vi "Alarm URL to Tag Name.vi"(11 "alarm URL":string="\\\\Nate-VM-LV2018\\Pfizer_FAST_20190409T090342\\Temperature.Alarms.Temperature:Lo") -> (3 "tag name":string)   [LabVIEW 2021, in "Dynamic Shared Variables.lvlib"]
uses:
  Dynamic Shared Variables.lvlib
  <vilib>/regexp/Match Regular Expression.xnode
panel:
  out "string after last '\\'.":string
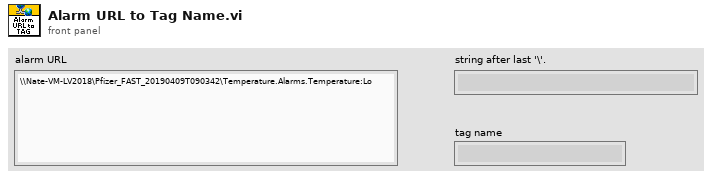
[diagram p1: front panel]
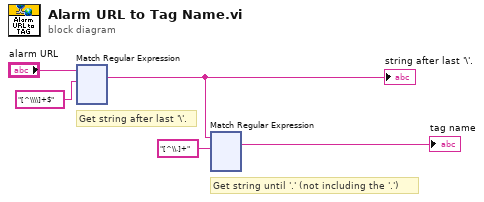
[diagram p0: block diagram]
diagram:
  # "Get string until '.' (not including the '.')"
  # "Get string after last '\\'."
  n1 = xnode "Match Regular Expression"("input string"="alarm URL", "regular expression"="[^\\\\]+$") -> ("whole match"=w3:string)  [unwired: 4 in, 4 out]
  "string after last '\\'." <- w3
  n2 = xnode "Match Regular Expression"("input string"=w3, "regular expression"="[^\\.]+") -> ("whole match"=→"tag name":string)  [unwired: 4 in, 4 out]
